vi "thcd401_set_unit.vi"(5 "unit":string="Magnet", 7 "channel":u8=1 min=1 max=4 step=1, 8 "error in":errorcluster, 11 "conn_id_in":refnum<k5>) -> (0 "error out":errorcluster, 3 "conn_id_out":refnum<k5>, 4 "status":bool)   [LabVIEW 2019]
panel:
  out "query":string
  # "7 chars at max"
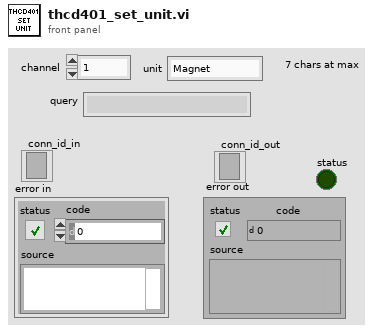
[diagram p1: front panel]
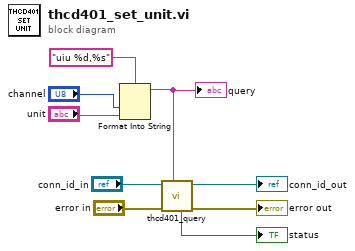
[diagram p0: block diagram]
diagram:
  n1 = Format Into String(format string="uiu %d,%s", "channel", "unit") -> (resulting string=w2:string)  [unwired: 2 in, 1 out]
  "query" <- w2
  n2 = call "thcd401_query.vi"("command"=w2, "error in"="error in", "conn_id_in"="conn_id_in") -> ("error out"=→"error out":errorcluster, "conn_id_out"=→"conn_id_out":refnum<k5>, "status"=→"status":bool)  [unwired: 5 in, 1 out]
